vi "CT_MagCurrent.vi"(0 "Coil Currents":waveform(dbl)[](graph)=[{"t0"=timestamp(3383307443.4356585 s since 1904-01-01), "dt"=0.0033333, "Y"=array[1000 elements], "attributes"=variant("NI_ChannelName"=variant(string "Current_CoilC"), "NI_UnitDescription"=variant(string "Volts"))}, {"t0"=timestamp(3383307443.4356723 s since 1904-01-01), "dt"=0.0033333, "Y"=array[1000 elements], "attributes"=variant("NI_ChannelName"=variant(string "Current_CoilB"), "NI_UnitDescription"=variant(string "Volts"))}, {"t0"=timestamp(3383307443.4356866 s since 1904-01-01), "dt"=0.0033333, "Y"=array[1000 elements], "attributes"=variant("NI_ChannelName"=variant(string "Current_CoilA"), "NI_UnitDescription"=variant(string "Volts"))}], 1 "Magnet Pulse Timing":dbl[](array[slide])=[-0.1, -0.2, -0.12] min=-2.0 max=0.0 scale=-2.0..0.0 scale format="%.3f") -> (2 "Coil D":i32=-4, 3 "Coil C":i32=-4, 4 "Coil B":i32=-2, 5 "Coil A":i32=-4)   [LabVIEW 2009]
uses:
  <vilib>/Analysis/NI_AALBase.lvlib
panel:
  in  "Magnet Pulse Timing 2":dbl[](array[slide])=[-0.1, -0.2, -0.12] min=-2.0 max=0.0 scale=-2.0..0.0 scale format="%.3f"
  in  "Magnet Pulse Timing":dbl[](array[slide])=[-0.1, -0.2, -0.12] min=-2.0 max=0.0 scale=-2.0..0.0 scale format="%.3f"
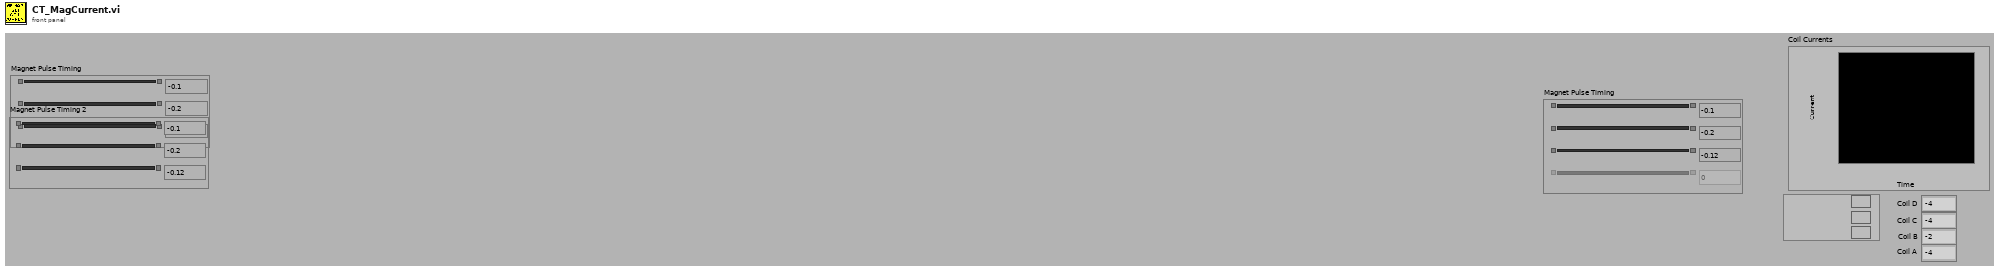
[diagram p1: front panel]
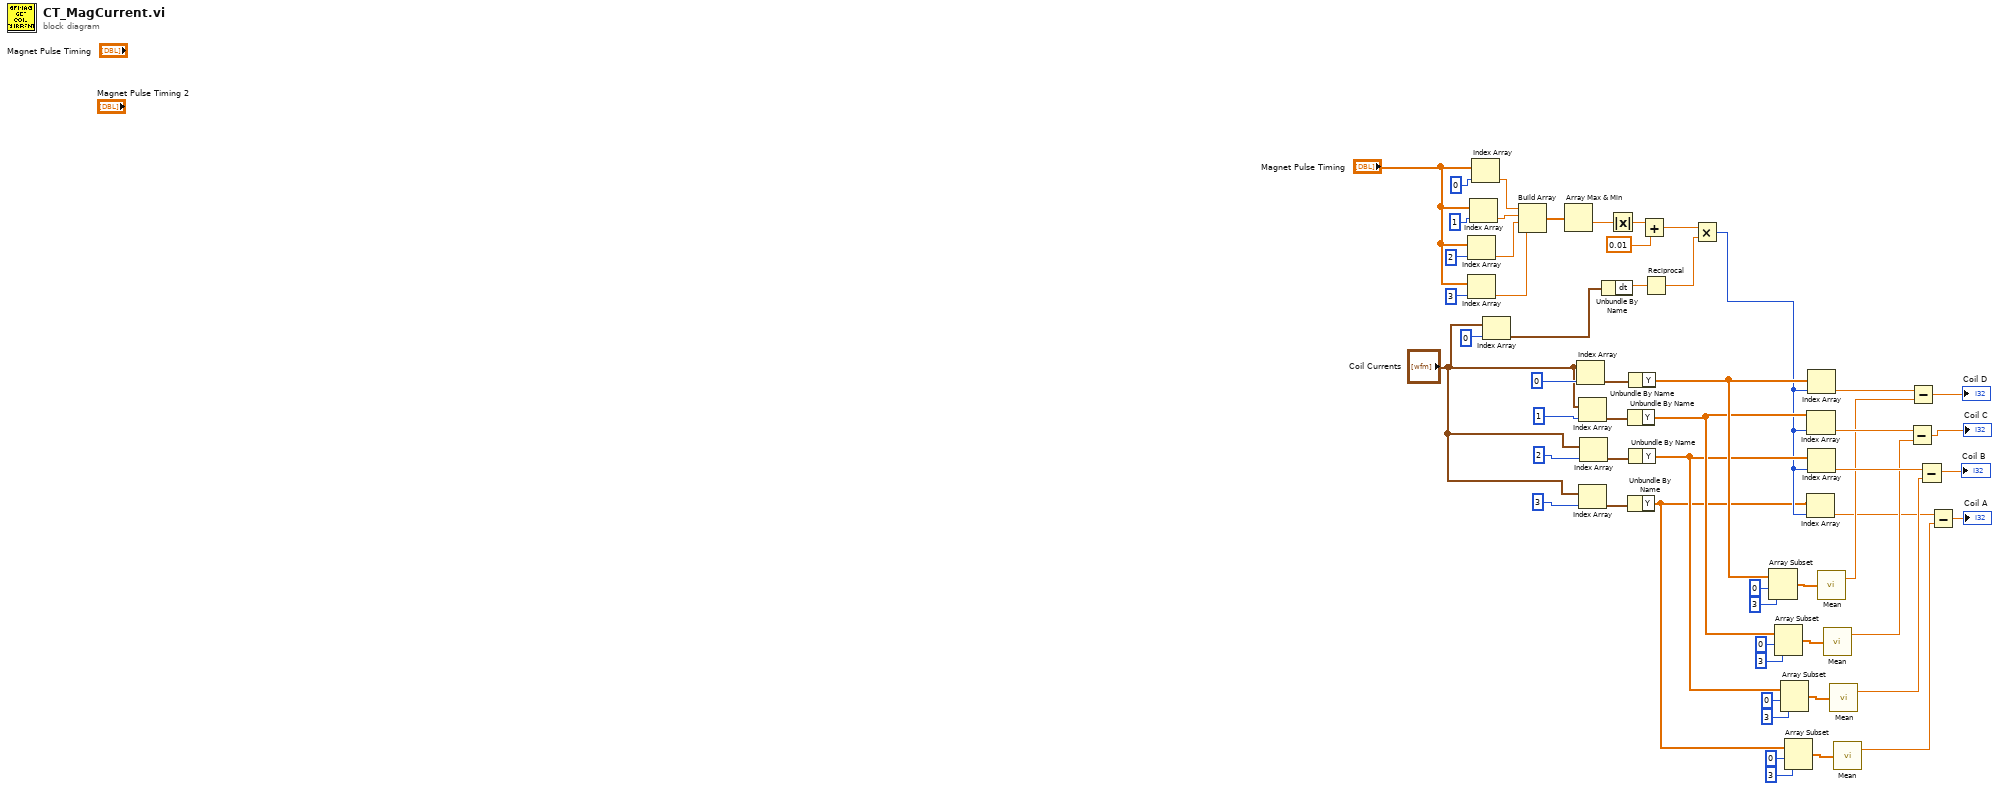
[diagram p0: block diagram]
diagram:
  n1 = Index Array(array="Magnet Pulse Timing", index=2) -> (element=w47:dbl)
  n2 = Index Array(array="Magnet Pulse Timing", index=3) -> (element=w15:dbl)
  n3 = Index Array(array="Magnet Pulse Timing", index=1) -> (element=w48:dbl)
  n4 = Index Array(array="Magnet Pulse Timing", index=0) -> (element=w49:dbl)
  n5 = Index Array(array="Coil Currents", index=0) -> (element=w22:waveform(dbl))
  n6 = Build Array(w49, w48, w47, w15) -> (w53:dbl[])
  n7 = Array Max & Min(array=w53) -> (min value=w52:dbl)  [unwired: 3 out]
  n8 = Index Array(array="Coil Currents", index=0) -> (element=w45:waveform(dbl))
  n9 = Index Array(array="Coil Currents", index=1) -> (element=w44:waveform(dbl))
  n10 = Index Array(array="Coil Currents", index=3) -> (element=w13:waveform(dbl))
  n11 = Index Array(array="Coil Currents", index=2) -> (element=w43:waveform(dbl))
  n12 = Unbundle By Name(w22) -> ("dt"=w21:dbl)
  n13 = Absolute Value(x=w52) -> (abs(x)=w50:dbl)
  n14 = Unbundle By Name(w44) -> ("Y"=w26:dbl[])
  n15 = Unbundle By Name(w13) -> ("Y"=w1:dbl[])
  n16 = Unbundle By Name(w45) -> ("Y"=w34:dbl[])
  n17 = Unbundle By Name(w43) -> ("Y"=w24:dbl[])
  n18 = Add(x=w50, y=0.01) -> (x+y=w20:dbl)
  n19 = Reciprocal(x=w21) -> (1/x=w19:dbl)
  n20 = Multiply(x=w20, y=w19) -> (x*y=w8:i32)
  n21 = Array Subset(array=w34, index=0, length=3) -> (w35:dbl[])
  n22 = Array Subset(array=w26, index=0, length=3) -> (w30:dbl[])
  n23 = Array Subset(array=w24, index=0, length=3) -> (w27:dbl[])
  n24 = Array Subset(array=w1, index=0, length=3) -> (w9:dbl[])
  n25 = Index Array(array=w1, index=w8) -> (element=w2:dbl)
  n26 = Index Array(array=w26, index=w8) -> (element=w41:dbl)
  n27 = Index Array(array=w34, index=w8) -> (element=w42:dbl)
  n28 = Index Array(array=w24, index=w8) -> (element=w40:dbl)
  n29 = call <vilib>:"Mean.vi"("X"=w35) -> ("mean"=w33:dbl)  [unwired: 1 out]
  n30 = call <vilib>:"Mean.vi"("X"=w30) -> ("mean"=w25:dbl)  [unwired: 1 out]
  n31 = call <vilib>:"Mean.vi"("X"=w27) -> ("mean"=w23:dbl)  [unwired: 1 out]
  n32 = call <vilib>:"Mean.vi"("X"=w9) -> ("mean"=w3:dbl)  [unwired: 1 out]
  n33 = Subtract(x=w41, y=w25) -> (x-y=→"Coil C":dbl)
  n34 = Subtract(x=w42, y=w33) -> (x-y=→"Coil D":dbl)
  n35 = Subtract(x=w40, y=w23) -> (x-y=→"Coil B":dbl)
  n36 = Subtract(x=w2, y=w3) -> (x-y=→"Coil A":dbl)
